vi "read config.vi"(8 "error in (no error)":errorcluster, 10 "config file path":path, 11 "USB IO in":refnum<class "USB IO.lvclass">) -> (0 "error out":errorcluster, 3 "USB IO out":refnum<class "USB IO.lvclass">)   [LabVIEW 2025, in "USB IO.lvlib" / "USB IO.lvclass"]
uses:
  USB IO.lvclass
  USB IO.lvclass/USB IO.ctl
  9b8b088c-8bc7-4bef-a6f3-163340907b3e.vi
  <vilib>/JDP Science/JSONtext/JSON text to Variant.vi
  <vilib>/JDP Science/JSONtext/LVClass Serializer/JSONtext LVClass Serializer.lvclass
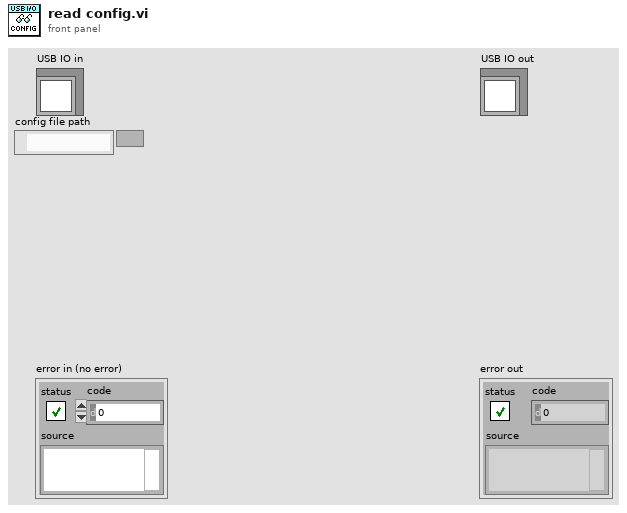
[diagram p1: front panel]
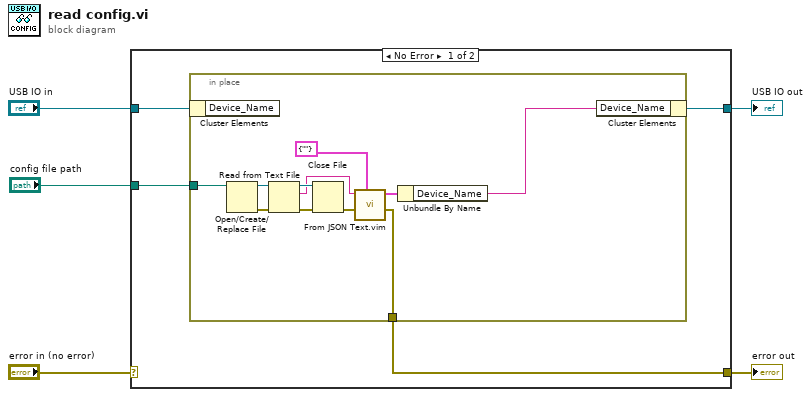
[diagram p0: block diagram]
diagram:
  n1 = case shown="No Error" "error in (no error)" {
    selector: "error in (no error)" -> [_ w22]
    tunnel: [w6 w22] -> w4
    tunnel: [w8 w21] -> w2
    tunnel: "USB IO in" -> [w9 w21]
    tunnel: "config file path" -> [w7 _]
    frame No Error {
      n2 = in-place {
        in-place-border: w7 -> [w14]
        in-place-border: [w10] -> w6
        n3 = in-place-cluster #1(w9) -> ()  [unwired: 1 out]
        n4 = Open/Create/Replace File(file path (use dialog)=w14) -> (refnum out=w17:refnum<file>, error out=w20:errorcluster)  [unwired: 5 in, 1 out]
        n5 = Read from Text File(file (use dialog)=w17, error in=w20) -> (refnum out=w18:refnum<file>, text=w16:string, error out=w19:errorcluster)  [unwired: 2 in, 1 out]
        n6 = Close File(refnum=w18, error in=w19) -> (error out=w15:errorcluster)  [unwired: 1 out]
        n7 = call "From JSON Text.vim"("Data Type and Default Value"=cluster{"Device_Name":string} {"Device_Name"=""}, "error in (no error)"=w15, "JSON"=w16) -> ("error out"=w10:errorcluster, "Data out"=w13:cluster{"Device_Name":string})  [unwired: 7 in]
        n8 = Unbundle By Name(w13) -> ("Device_Name"=w11:string)
        n9 = in-place-cluster #1("Device_Name"=w11) -> (w8:refnum<class "USB IO.lvclass">)
      }
    }
    frame Error {
    }
  }
  "error out" <- w4
  "USB IO out" <- w2
